vi "7-4.vi"() -> ()   [LabVIEW 2017]
panel:
  in  "停止":bool
  in  "显示或隐藏":bool
  out "波形图":dbl[](graph)
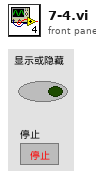
[diagram p1: front panel]
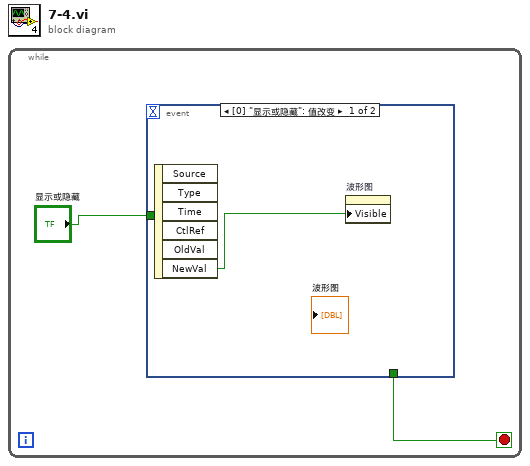
[diagram p0: block diagram]
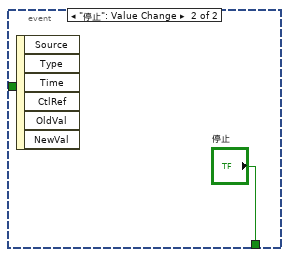
[diagram p2: hidden frame]
diagram:
  n1 = while {
    stop <- w1 stop-if-true
    n2 = event shown="[0] \"显示或隐藏\": 值改变" {
      selector: _ -> [_ _]
      dyn-events: _ -> [_ _]
      timeout: _ -> [_ _]
      tunnel: "显示或隐藏" -> [_ _]
      tunnel: [_ "停止"] -> w1
      event "显示或隐藏": Value Change {
        n3 = event-data() -> ("NewVal"=w3:bool)  [unwired: 1 in, 5 out]
        n4 = property on="波形图" class="WFGraph (严格)"("Visible"=w3) -> ()  [unwired: 2 in, 2 out]
      }
      event "停止": Value Change {
        n5 = event-data() -> ()  [unwired: 1 in, 6 out]
      }
    }
  }
